vi "Initialize.vi"(8 "error in (no error)":errorcluster, 11 "VICI Settings":T1) -> (0 "error out":errorcluster, 1 "Initialized":bool, 2 "No Pump Connected":bool, 3 "VICI Settings":T1)   [LabVIEW 2018, in "VICI M6 M50 Party Mode.lvlib"]
uses:
  VICI M6 M50 Party Mode.lvlib
  Settings Cluster.ctl
  <vilib>/Instr/_visa.llb/VISA Flush IO Buffer Mask.ctl
  <vilib>/Instr/_visa.llb/VISA Configure Serial Port (Instr).vi
  VICI Global Library.lvlib
panel:
  out "Bytes at Port 2":u32
  out "Bytes at Port":u32
  out "read buffer 5":string
  out "read buffer 4":string
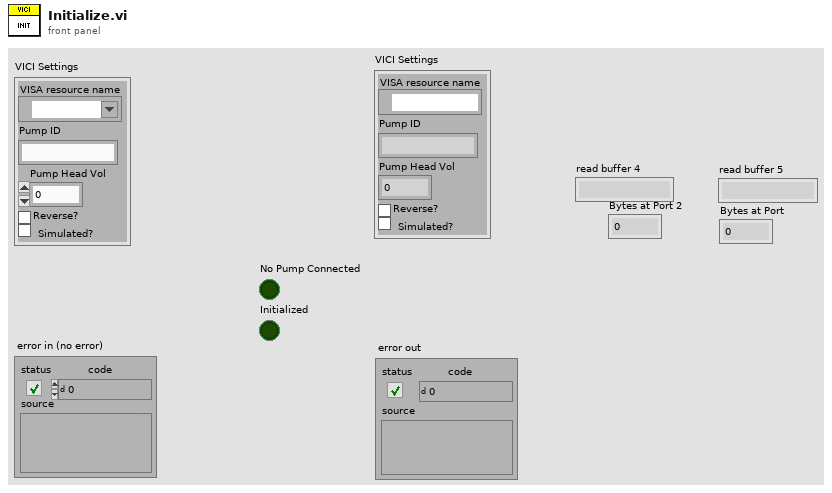
[diagram p1: front panel]
types:
  T1 = typedef "VICI M6 M50 Party Mode.lvlib/Settings Cluster.ctl" = cluster{"VISA resource name":refnum<visa-resource-name>, "Pump ID":string, "Pump Head Vol":dbl, "Reverse?":bool, "Simulated?":bool}
  T2 = typedef "VICI M6 M50 Party Mode.lvlib/VICI Global Library.lvlib/VICI Global.ctl" = cluster{"Busy":bool, "VISA #":string, "Current Pump":string, "Current Function":string, "Pump Array":string[], "Last Success":timestamp, "ID Queue":string[]}
  T3 = typedef "VISA Flush IO Buffer Mask.ctl" = u16
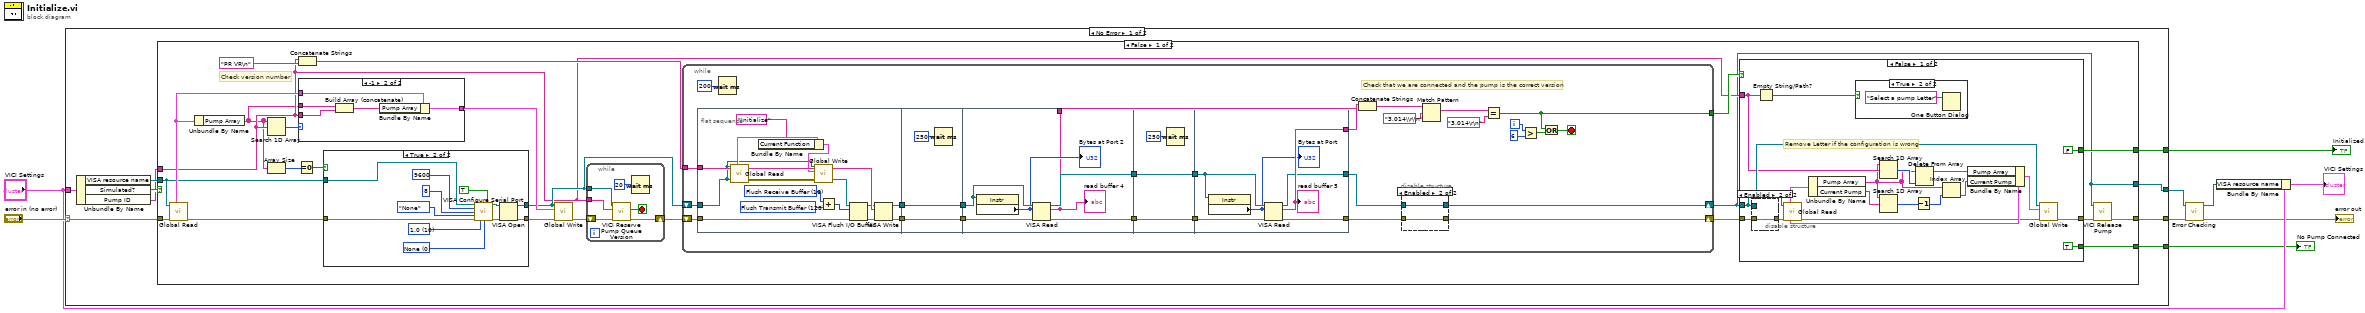
[diagram p0: block diagram]
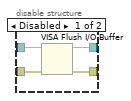
[diagram p2: hidden frame]
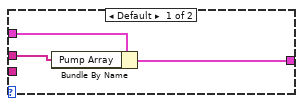
[diagram p4: hidden frame]
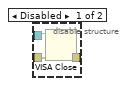
[diagram p5: hidden frame]
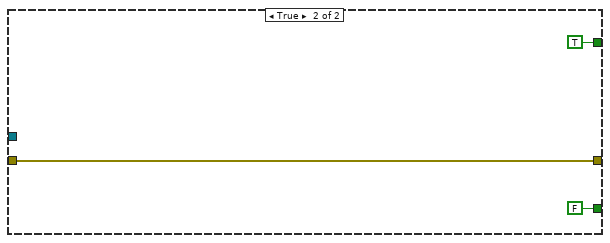
[diagram p7: hidden frame]
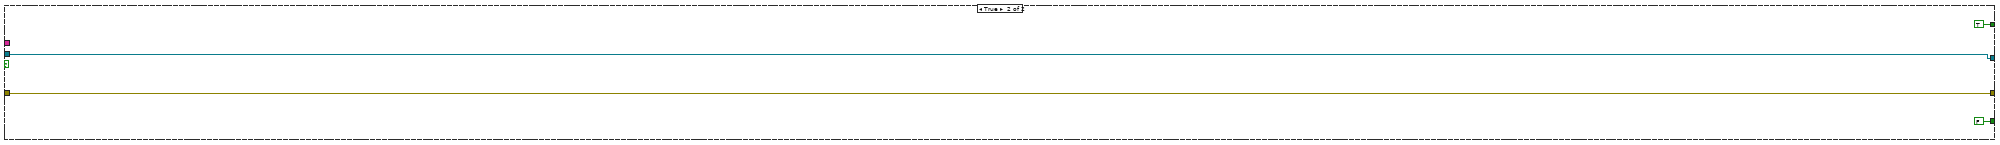
[diagram p8: hidden frame]
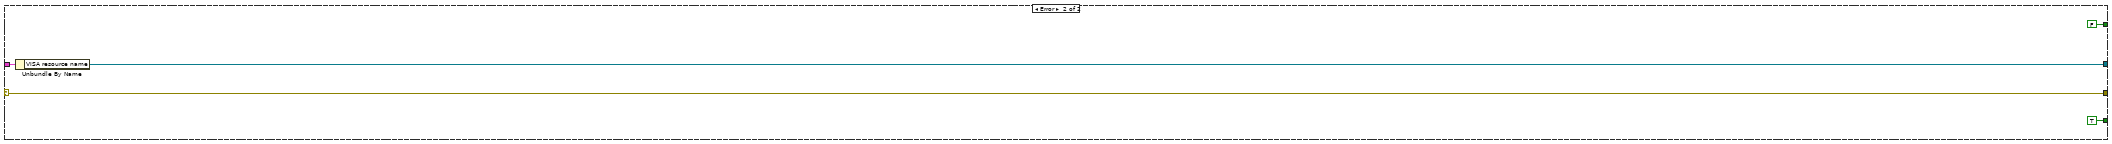
[diagram p9: hidden frame]
diagram:
  n1 = case shown="No Error" "error in (no error)" {
    selector: "error in (no error)" -> [w18 w169]
    tunnel: "VICI Settings" -> [w15 w168]
    tunnel: [w16 w169] -> w5
    tunnel: [w13 w167] -> w6
    tunnel: [w11 FALSE] -> w4
    tunnel: [w10 TRUE] -> w3
    frame No Error {
      n2 = Unbundle By Name(w15) -> ("VISA resource name"=w14:refnum<visa-resource-name>, "Simulated?"=w17:bool, "Pump ID"=w12:string)
      n3 = case shown="False" w17 {
        tunnel: w18 -> [w24 w164]
        tunnel: [w26 w164] -> w16
        tunnel: [w27 w163] -> w13
        tunnel: w14 -> [w25 w163]
        tunnel: w12 -> [w30 _]
        tunnel: [w39 TRUE] -> w11
        tunnel: [w36 FALSE] -> w10
        frame False {
          # "Check version number"
          n4 = call "Global Read.vi"("VISA #"=w25, "error in (no error)"=w24) -> ("Global for this VISA"=w33:T2, "error out"=w23:errorcluster)  [unwired: 2 in, 5 out]
          n5 = Unbundle By Name(w33) -> ("Pump Array"=w21:string[])
          n6 = Search 1D Array(1D array=w21, element=w30) -> (index of element=w29:i32)  [unwired: 1 in]
          n7 = Array Size(array=w21) -> (size(s)=w20:i32)
          n8 = Equal To 0?(x=w20) -> (x = 0?=w19:bool)
          n9 = Concatenate Strings(w30, "PR VR\n" ("string")) -> (w37:string)
          n10 = case shown="-1" w29 {
            tunnel: [w121 w127] -> w34
            tunnel: w33 -> [w123 w126]
            tunnel: w21 -> [w122 w125]
            tunnel: w30 -> [_ w124]
            frame Default {
              n11 = Bundle By Name(cluster=w123, "Pump Array"=w122) -> (w121:T2)
            }
            frame -1 {
              n12 = Build Array (concatenate)(w125, w124) -> (w128:string[])
              n13 = Bundle By Name(cluster=w126, "Pump Array"=w128) -> (w127:T2)
            }
          }
          n14 = case shown="True" w19 {
            tunnel: [w107 w112] -> w31
            tunnel: w25 -> [w107 w111]
            tunnel: w23 -> [w108 w110]
            tunnel: [w108 w109] -> w22
            frame False {
            }
            frame True {
              w116 = u16 0 items=["None", "XON/XOFF", "RTS/CTS", "XON/XOFF & RTS/CTS", "DTR/DSR", "XON/XOFF & DTR/DSR"] ("flow control (0:none)")
              w117 = u16 10 items=["1.0"=10, "1.5"=15, "2.0"=20] ("stop bits (10: 1 bit)")
              n15 = call-poly "VISA Configure Serial Port"("VISA resource name"=w111, "Enable Termination\nChar (T)"=TRUE ("Enable Termination\nChar (T)"), "baud rate (9600)"=u32 9600, "data bits (8)"=u16 8, "parity (0:none)"=enum16{"None", "Odd", "Even", "Mark", "Space"}."None", "error in (no error)"=w110, "stop bits (10: 1 bit)"=w117, "flow control (0:none)"=w116) -> ("VISA resource name out"=w114:refnum<visa-resource-name>, "error out"=w115:errorcluster)  [unwired: 6 in]
              n16 = VISA Open(error in (no error)=w115, VISA resource name=w114) -> (VISA resource name=w112:refnum<visa-resource-name>, error out=w109:errorcluster)  [unwired: 3 in]
            }
          }
          n17 = call "Global Write.vi"("error in (no error)"=w22, "VICI Global"=w34, "VISA # in"=w31) -> ("error out"=w32:errorcluster)  [unwired: 7 in, 1 out]
          n18 = while {
            tunnel: w31 -> [w133]
            tunnel: w30 -> [w132]
            shift-right: [w130] -> w35
            shift-left: w32 -> [w131]
            stop <- w129 stop-if-true
            n19 = call "VICI Reserve Pump Queue Version.vi"("error in (no error)"=w131, "Pump ID"=w132, "VISA # in"=w133) -> ("error out"=w130:errorcluster, "Loop Completed"=w129:bool)  [unwired: 6 in, 1 out]
            n20 = Wait (ms)(milliseconds to wait=u32 20) -> ()  [unwired: 1 out]
          }
          n21 = while {
            tunnel: [w46] -> w41
            tunnel: w37 -> [w58]
            shift-right: [w59] -> w40
            shift-left: w35 -> [w52]
            shift-right: [w50] -> w27
            shift-left: w31 -> [w51]
            i -> [w49]
            stop <- w45 stop-if-true
            # "Check that we are connected and the pump is the correct version"
            n22 = flat-sequence {
              tunnel: w52 -> [w84]
              tunnel: w51 -> [w75]
              tunnel: w58 -> [w88]
              tunnel: [w81] -> w42
              tunnel: [w80] -> w43
              tunnel: [w89] -> w68
              tunnel: w43 -> [w89]
              tunnel: w42 -> [w90]
              tunnel: [w90] -> w67
              tunnel: w68 -> [w94]
              tunnel: w67 -> [w97]
              tunnel: [w96] -> w66
              tunnel: [w95] -> w65
              tunnel: [w92] -> w54
              tunnel: w66 -> [w100]
              tunnel: [w100] -> w64
              tunnel: w65 -> [w99]
              tunnel: [w99] -> w63
              tunnel: w64 -> [w106]
              tunnel: w63 -> [w102]
              tunnel: [w105] -> w60
              tunnel: [w104] -> w55
              tunnel: [w103] -> w61
              frame #0 {
                w86 = T3 128 items=["Flush Receive Buffer"=16, "Write Transmit Buffer to Device"=32, "Flush Receive Buffer (No I/O)"=64, "Flush Transmit Buffer"=128] ("Mask")
                w87 = T3 16 items=["Flush Receive Buffer"=16, "Write Transmit Buffer to Device"=32, "Flush Receive Buffer (No I/O)"=64, "Flush Transmit Buffer"=128] ("Mask")
                n23 = call "Global Read.vi"("VISA #"=w75) -> ("Global for this VISA"=w78:T2, "error out"=w79:errorcluster)  [unwired: 3 in, 5 out]
                n24 = Bundle By Name(cluster=w78, "Current Function"="Initialize") -> (w77:T2)
                n25 = call "Global Write.vi"("error in (no error)"=w79, "VICI Global"=w77, "VISA # in"=w75) -> ()  [unwired: 7 in, 2 out]
                n26 = Add(x=w87, y=w86) -> (x+y=w85:T3)
                n27 = VISA Flush I/O Buffer(VISA resource name=w75, mask (16)=w85, error in (no error)=w84) -> (VISA resource name out=w83:refnum<visa-resource-name>, error out=w82:errorcluster)
                n28 = VISA Write(VISA resource name=w83, write buffer=w88, error in (no error)=w82) -> (VISA resource name out=w80:refnum<visa-resource-name>, error out=w81:errorcluster)  [unwired: 1 out]
              }
              frame #1 {
                n29 = Wait (ms)(milliseconds to wait=u32 250) -> ()  [unwired: 1 out]
              }
              frame #2 {
                n30 = property class="Instr"(reference=w94) -> ("Serial Settings:Number of Bytes at Serial Port"=w93:u32)  [unwired: 1 in, 2 out]
                "Bytes at Port 2" <- w93
                n31 = VISA Read(VISA resource name=w94, byte count=w93, error in (no error)=w97) -> (VISA resource name out=w95:refnum<visa-resource-name>, read buffer=w92:string, error out=w96:errorcluster)  [unwired: 1 out]
                "read buffer 4" <- w92
              }
              frame #3 {
                n32 = Wait (ms)(milliseconds to wait=u32 250) -> ()  [unwired: 1 out]
              }
              frame #4 {
                n33 = property class="Instr"(reference=w102) -> ("Serial Settings:Number of Bytes at Serial Port"=w101:u32)  [unwired: 1 in, 2 out]
                "Bytes at Port" <- w101
                n34 = VISA Read(VISA resource name=w102, byte count=w101, error in (no error)=w106) -> (VISA resource name out=w103:refnum<visa-resource-name>, read buffer=w104:string, error out=w105:errorcluster)  [unwired: 1 out]
                "read buffer 5" <- w104
              }
            }
            n35 = Wait (ms)(milliseconds to wait=u32 200) -> ()  [unwired: 1 out]
            n36 = Concatenate Strings(w55, w54) -> (w53:string)
            n37 = disable-structure shown="Enabled" {
              disable-tunnel: w61 -> [w72 w73]
              disable-tunnel: w60 -> [w71 w74]
              disable-tunnel: [w70 w74] -> w59
              disable-tunnel: [w69 w73] -> w50
              frame Disabled {
                n38 = VISA Flush I/O Buffer(VISA resource name=w72, error in (no error)=w71) -> (VISA resource name out=w69:refnum<visa-resource-name>, error out=w70:errorcluster)  [unwired: 1 in]
              }
              frame Enabled {
              }
            }
            n39 = Match Pattern(string=w53, regular expression="3.014\\r\\n") -> (match substring=w56:string)  [unwired: 1 in, 3 out]
            n40 = Equal?(x=w56, y="3.014\r\n") -> (x = y?=w46:bool)
            n41 = Greater?(x=w49, y=6) -> (0:w44:bool)
            n42 = Or(x=w46, y=w44) -> (x .or. y?=w45:bool)
          }
          n43 = case shown="False" w41 {
            tunnel: w27 -> [w146 _]
            tunnel: w40 -> [w152 w158]
            tunnel: [TRUE FALSE] -> w36
            tunnel: [w140 w158] -> w28
            tunnel: [FALSE TRUE] -> w39
            tunnel: w30 -> [w144 _]
            frame False {
              # "Remove Letter if the configuration is wrong"
              n44 = disable-structure shown="Enabled" {
                disable-tunnel: w152 -> [w155 w156]
                disable-tunnel: w146 -> [w154 _]
                disable-tunnel: [w153 w156] -> w145
                frame Disabled {
                  n45 = VISA Close(VISA resource name=w154, error in (no error)=w155) -> (error out=w153:errorcluster)
                }
                frame Enabled {
                }
              }
              n46 = Empty String/Path?(string/path=w144) -> (empty?=w149:bool)
              n47 = call "Global Read.vi"("VISA #"=w146, "error in (no error)"=w145) -> ("Global for this VISA"=w148:T2, "error out"=w147:errorcluster)  [unwired: 2 in, 5 out]
              n48 = Unbundle By Name(w148) -> ("Pump Array"=w139:string[], "Current Pump"=w138:string)
              n49 = case shown="True" w149 {
                frame False {
                }
                frame True {
                  n50 = One Button Dialog(message="Select a pump Letter") -> ()  [unwired: 1 in, 1 out]
                }
              }
              n51 = Search 1D Array(1D array=w139, element=w144) -> (index of element=w143:i32)  [unwired: 1 in]
              n52 = Search 1D Array(1D array=w139, element=w138) -> (index of element=w137:i32)  [unwired: 1 in]
              n53 = Decrement(x=w137) -> (x-1=w136:i32)
              n54 = Delete From Array(array=w139, index=w143) -> (array with subset deleted=w141:string[])  [unwired: 1 in, 1 out]
              n55 = Index Array(array=w139, index=w136) -> (element=w135:string)
              n56 = Bundle By Name(cluster=w148, "Pump Array"=w141, "Current Pump"=w135) -> (w142:T2)
              n57 = call "Global Write.vi"("error in (no error)"=w147, "VICI Global"=w142, "VISA # in"=w146) -> ("error out"=w140:errorcluster)  [unwired: 7 in, 1 out]
            }
            frame True {
            }
          }
          n58 = call "VICI Release Pump.vi"("error in (no error)"=w28, "VISA # in"=w27) -> ("error out"=w26:errorcluster)  [unwired: 8 in, 1 out]
        }
        frame True {
        }
      }
    }
    frame Error {
      n59 = Unbundle By Name(w168) -> ("VISA resource name"=w167:refnum<visa-resource-name>)
    }
  }
  "Initialized" <- w4
  "No Pump Connected" <- w3
  n60 = call "Error Checking.vi"("error in (no error)"=w5, "VISA resource name"=w6) -> ("error out"=→"error out":errorcluster, "VISA resource name"=w2:refnum<visa-resource-name>)  [unwired: 7 in, 1 out]
  n61 = Bundle By Name(cluster="VICI Settings", "VISA resource name"=w2) -> (→"VICI Settings":T1)
